vi "APS set field bus trigger param.vi"(6 "Param_Val":i32, 7 "Param_No":i32, 8 "error in (no error)":errorcluster caption="错误输入（无错误）", 9 "MOD_No":i32, 10 "BUS_No":i32, 11 "Board_ID":i32) -> (0 "error out":errorcluster caption="错误输出", 3 "function return":i32)   [LabVIEW 2011, in "APS168.lvlib"]
doc: "I32 FNTYPE APS_set_field_bus_trigger_param( I32 Board_ID, I32 BUS_No, I32 MOD_No, I32 Param_No, I32 Param_Val );"
uses:
  APS168.lvlib
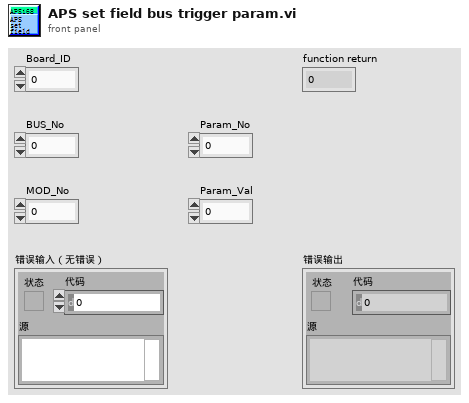
[diagram p1: front panel]
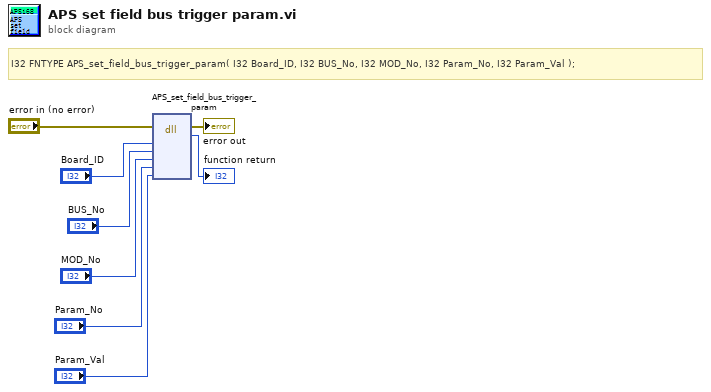
[diagram p0: block diagram]
diagram:
  # "I32 FNTYPE APS_set_field_bus_trigger_param( I32 Board_ID, I32 BUS_No, I32 MOD_No, I32 Param_No, I32 Param_Val );"
  n1 = dll-call lib="PTH1Labs E软件ADLINK 204CAPS_1_7_1_LIB line 连续运动204APS168.*" fn="APS_set_field_bus_trigger_param"(error in="error in (no error)", "Board_ID"="Board_ID", "BUS_No"="BUS_No", "MOD_No"="MOD_No", "Param_No"="Param_No", "Param_Val"="Param_Val") -> (error out=→"error out":errorcluster, →"function return":i32)  [unwired: 7 in, 1 out]
